vi "Write outputs.vi"(5 "outputs":string[](array[string]), 9 "TestCase in":refnum<class "TestCase.lvclass">) -> (3 "TestCase out":refnum<class "TestCase.lvclass">)   [LabVIEW 2014, in "TestCase.lvclass"]
uses:
  TestCase.lvclass
  TestCase.lvclass/TestCase.ctl
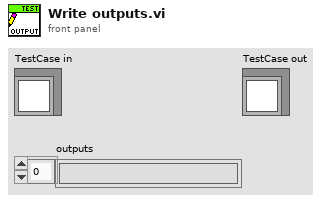
[diagram p1: front panel]
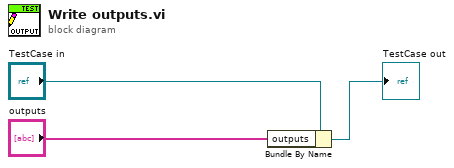
[diagram p0: block diagram]
diagram:
  n1 = Bundle By Name(cluster="TestCase in", "outputs"="outputs") -> (→"TestCase out":refnum<class "TestCase.lvclass">)
